vi "Ping.vi"(7 "Ack Timeout":i32=200, 8 "error in":errorcluster) -> (0 "error out":errorcluster, 1 "Response":string, 3 "Timed Out":bool)   [LabVIEW 2015, in "Generic Module Library.lvlib" / "Template G_Module.lvlib"]
uses:
  Template G_Module.lvlib
  Private Controls/Module Message Cluster Components/Message Data Cluster.ctl
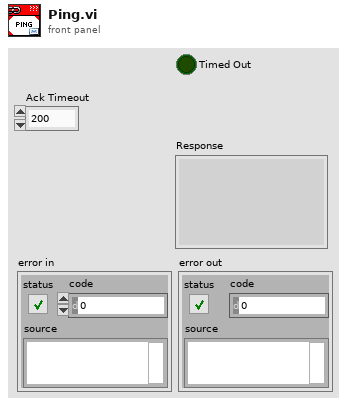
[diagram p1: front panel]
types:
  T1 = typedef "Generic Module Library.lvlib/Template G_Module.lvlib/Message Data Cluster.ctl" = cluster{"Module Action":string, "Message Data":variant}
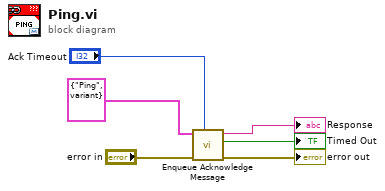
[diagram p0: block diagram]
diagram:
  n1 = call "Enqueue Acknowledge Message.vi"("Ack Timeout"="Ack Timeout", "error in"="error in", "Message Data"=T1 {"Module Action"="Ping", "Message Data"=variant}) -> ("error out"=→"error out":errorcluster, "Timed Out"=→"Timed Out":bool, "Response Data"=→"Response":string)  [unwired: 6 in]
